vi "Sensor Load File.vi"(8 "error in (no error)":errorcluster caption="错误输入（无错误）", 10 "pszFilename":string, 11 "sensorHandle":i32) -> (0 "error out":errorcluster caption="错误输出", 2 "pszFilename out":string, 3 "function return":i32)   [LabVIEW 2018]
doc: "extern int __stdcall APSxSensorLoadFile (int sensorHandle, IN char * pszFilename);"
uses:
  APSx.dll/APSx.dll
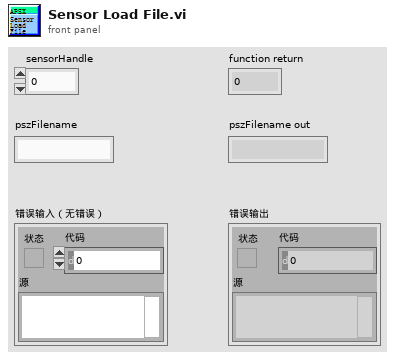
[diagram p1: front panel]
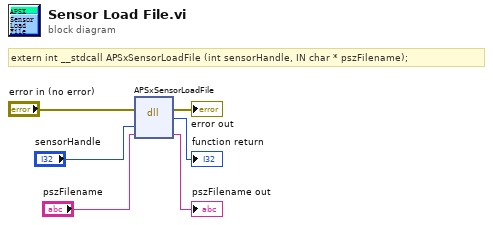
[diagram p0: block diagram]
diagram:
  # "extern int __stdcall APSxSensorLoadFile (int sensorHandle, IN char * pszFilename);"
  n1 = dll-call lib="PTH2[abs D项目Feng恒隆项目Labview传感器对中台SourcesAPSx.dllAPSx.*" fn="APSxSensorLoadFile"(error in="error in (no error)", "sensorHandle"="sensorHandle", "pszFilename"="pszFilename") -> (error out=→"error out":errorcluster, →"function return":i32, "pszFilename"=→"pszFilename out":string)  [unwired: 3 in, 1 out]
